vi "Variant_BuildArrayFromFlattenedData.vi"(8 "error in (no error)":errorcluster, 9 "Flattened Elements":string[](array[string]), 10 "Dimensions":u32[](array[numeric]), 11 "Default Array":variant) -> (0 "error out":errorcluster, 3 "Output Array":variant)   [LabVIEW 2013]
uses:
  <vilib>/Utility/GetType.llb/Type Descriptor I16.ctl
  TypeDescriptor/TypeDescriptor_GetType.vi
  TypeDescriptor/TypeDescriptor_GetPString.vi
  <vilib>/Utility/GetType.llb/Get Type Code from I16 Array And Pos.vi
  <vilib>/Utility/GetType.llb/TD_Get Array Information.vi
  TypeDescriptor/TypeDescriptor_SetName.vi
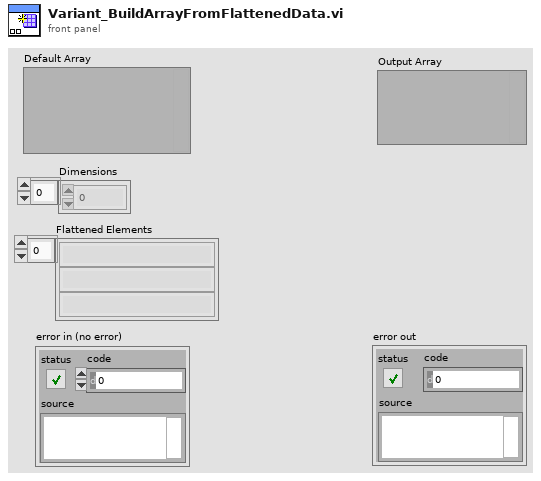
[diagram p1: front panel]
types:
  T1 = typedef "Type Descriptor I16.ctl" = i16
  T2 = typedef "Type Descriptor I16 Array.ctl" = T1[]
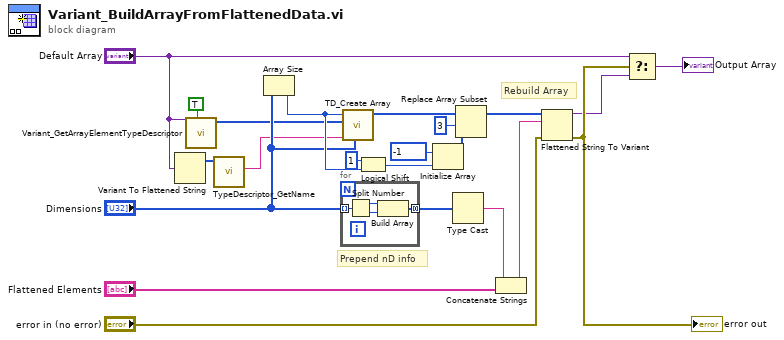
[diagram p0: block diagram]
diagram:
  # "Prepend nD info"
  # "Rebuild Array"
  n1 = Variant To Flattened String(Variant="Default Array") -> (1:w3:i16[])  [unwired: 1 out]
  n2 = call "Variant_GetArrayElementTypeDescriptor.vi"("Name Element if empty string (F)"=TRUE, "Array"="Default Array") -> ("Element Descriptor"=w5:i16[])  [unwired: 8 in, 1 out]
  n3 = call "TypeDescriptor_GetName.vi"("type descriptor"=w3) -> ("name"=w1:string)  [unwired: 8 in, 2 out]
  n4 = Array Size(array="Dimensions") -> (size(s)=w22:i32)
  n5 = for {
    tunnel: "Dimensions" -> [w26] mode=indexing
    tunnel: [w23] -> w15 mode=concatenating
    n6 = Split Number(x=w26) -> (hi(x)=w25:u16, lo(x)=w24:u16)
    n7 = Build Array(w25, w24) -> (w23:u16[])
  }
  n8 = call <vilib>:"TD_Create Array.vi"("Dim Lengths"="Dimensions", "Name"=w1, "Array Elt"=w5, "N Dims"=w22) -> ("NewArray"=w11:T2)  [unwired: 7 in]
  n9 = Logical Shift(y=i16 1, x=w22) -> (x << y=w18:i32)
  n10 = Initialize Array(T1 -1 ("Numeric"), w18) -> (w14:T1[])
  n11 = Type Cast(x=w15) -> (*(type *) &x=w16:string)  [unwired: 1 in]
  n12 = Replace Array Subset(array=w11, new element=w14, index=3) -> (w12:T2)
  n13 = Concatenate Strings(w16, "Flattened Elements") -> (w20:string)
  n14 = Flattened String To Variant(4:"error in (no error)", 6:w20, 7:w12) -> (0:w8:errorcluster, 3:w7:variant)
  "error out" <- w8
  n15 = Select(t="Default Array", s=w8, f=w7) -> (s? t:f=→"Output Array":variant)
